vi "Drive_Get_Speed.vi"() -> (0 "LeftSpeed":dbl, 3 "RightSpeed":dbl)   [LabVIEW 2020]
uses:
  DriveGlobals.vi
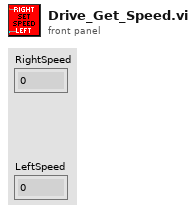
[diagram p1: front panel]
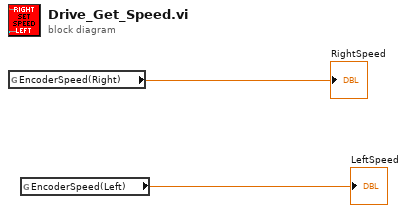
[diagram p0: block diagram]
diagram:
  n1 = global read "DriveGlobals.vi" "EncoderSpeed(Right)"() -> (→"RightSpeed":dbl)
  n2 = global read "DriveGlobals.vi" "EncoderSpeed(Left)"() -> (→"LeftSpeed":dbl)
